vi "Log Display Ref.vi"(8 "error in":errorcluster, 11 "log display ref":refnum<vi>) -> (0 "error out":errorcluster, 3 "log display ref out":refnum<vi>)   [LabVIEW 2014, in "lvprj2html.lvlib"]
uses:
  lvprj2html.lvlib
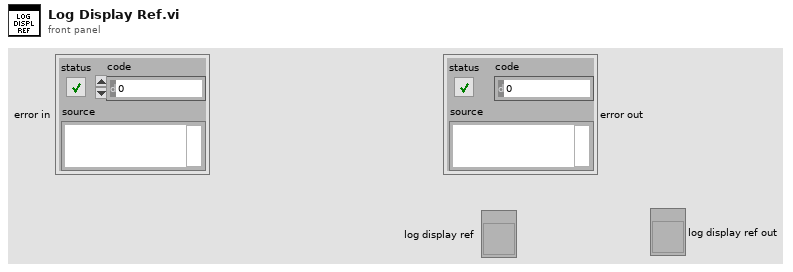
[diagram p1: front panel]
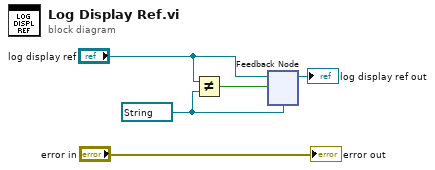
[diagram p0: block diagram]
diagram:
  w5 = refnum<vi> refnum ("log display")
  n1 = Not Equal?(x="log display ref", y=w5) -> (x != y?=w3:bool)
  n2 = feedback #1(w5) -> (→"log display ref out":refnum<vi>)
  n3 = feedback-in #1("log display ref", w3) -> ()
  "error out" <- "error in"
